vi "MIPI_RFEE_Create Patterns and save to HWS file_Wo_SetID.vi"(1 "Write Data":cluster{"USID":u8, "Register":u8, "Data":u8} {"Register" format="%.0x"; "USID" max=15 format="%.0x"}, 2 "Mode":enum16{"Write", "Read"}(ring), 5 "file path":path=path "C:/Users/user/Documents/AD2240/Waveforms/RFFE6", 12 "Save .HWS?":bool, 13 "Filename":string) -> ()   [LabVIEW 2013]
doc: "This VI demonstaits how to write to and read back data from a MIPI device. To run this VI:\n1) Change Resource name to the name of your HSDIO card\n2) The MIPI clock will run at <Sample Clock Rate>/<Oversample Factor>. This is 26 MHz (full rate). If your device should be run at a slower rate, decrease the sample clock rate and (or) increase the oversample rate.\n3. At 104MHz, the RTD value should be ~5 for a 1.5 meter cable. If you are running at a different clock rate or using a different length cable, adjust the RTD Compensation value so the MIPI data is stable at the falling edge of the clock. If you need futher timing adjustment, consider setting the data position to \"Delay from Sample Clock Rising Edge\" and configuring this delay."
uses:
  MIPI_RFFE/Ctrls/RegReadWrite.ctl
  MIPI_RFFE/Ctrls/Configuration.ctl
  MIPI_RFFE/Ctrls/ClockDataChannels.ctl
  MIPI_RFFE/Ctrls/ExtendedRegReadWrite.ctl
panel:
  out "Digital Waveform Graph":digitalwaveform(graph)={"t0"=timestamp(3585852840.1106524 s since 1904-01-01), "dt"=5e-07, "Y"={"transitions"=[], "data"=[[1, 0, 1, 0], [1, 0, 1, 0], [1, 0, 1, 0], [1, 0, 1, 0], [1, 0, 1, 0], [1, 0, 1, 0], [1, 0, 1, 0], [1, 0, 1, 0], [0, 0, 0, 0], [0, 0, 0, 0], [0, 0, 0, 0], [0, 0, 0, 0], [0, 0, 0, 0], [0, 0, 0, 0], [0, 0, 0, 0], [0, 0, 0, 0], [0, 1, 0, 1], [0, 1, 0, 1], [0, 1, 0, 1], [0, 1, 0, 1], [0, 0, 0, 0], [0, 0, 0, 0], [0, 0, 0, 0], [0, 0, 0, 0], [1, 1, 1, 1], [1, 1, 1, 1], [1, 1, 1, 1], [1, 1, 1, 1], [1, 0, 1, 0], [1, 0, 1, 0], [1, 0, 1, 0], [1, 0, 1, 0], [1, 1, 1, 1], [1, 1, 1, 1], [1, 1, 1, 1], [1, 1, 1, 1], [1, 0, 1, 0], [1, 0, 1, 0], [1, 0, 1, 0], [1, 0, 1, 0], [0, 1, 0, 1], [0, 1, 0, 1], [0, 1, 0, 1], [0, 1, 0, 1], [0, 0, 0, 0], [0, 0, 0, 0], [0, 0, 0, 0], [0, 0, 0, 0], [0, 1, 0, 1], [0, 1, 0, 1], [0, 1, 0, 1], [0, 1, 0, 1], [0, 0, 0, 0], [0, 0, 0, 0], [0, 0, 0, 0], [0, 0, 0, 0], [1, 1, 1, 1], [1, 1, 1, 1], [1, 1, 1, 1], [1, 1, 1, 1], [1, 0, 1, 0], [1, 0, 1, 0], [1, 0, 1, 0], [1, 0, 1, 0], [0, 1, 0, 1], [0, 1, 0, 1], [0, 1, 0, 1], [0, 1, 0, 1], [0, 0, 0, 0], [0, 0, 0, 0], [0, 0, 0, 0], [0, 0, 0, 0], [1, 1, 1, 1], [1, 1, 1, 1], [1, 1, 1, 1], [1, 1, 1, 1], [1, 0, 1, 0], [1, 0, 1, 0], [1, 0, 1, 0], [1, 0, 1, 0], [1, 1, 1, 1], [1, 1, 1, 1], [1, 1, 1, 1], [1, 1, 1, 1], [1, 0, 1, 0], [1, 0, 1, 0], [1, 0, 1, 0], [1, 0, 1, 0], [1, 1, 1, 1], [1, 1, 1, 1], [1, 1, 1, 1], [1, 1, 1, 1], [1, 0, 1, 0], [1, 0, 1, 0], [1, 0, 1, 0], [1, 0, 1, 0], [0, 1, 0, 1], [0, 1, 0, 1], [0, 1, 0, 1], [0, 1, 0, 1], [0, 0, 0, 0], [0, 0, 0, 0], [0, 0, 0, 0], [0, 0, 0, 0], [0, 1, 0, 1], [0, 1, 0, 1], [0, 1, 0, 1], [0, 1, 0, 1], [0, 0, 0, 0], [0, 0, 0, 0], [0, 0, 0, 0], [0, 0, 0, 0], [1, 1, 1, 1], [1, 1, 1, 1], [1, 1, 1, 1], [1, 1, 1, 1], [1, 0, 1, 0], [1, 0, 1, 0], [1, 0, 1, 0], [1, 0, 1, 0], [1, 1, 1, 1], [1, 1, 1, 1], [1, 1, 1, 1], [1, 1, 1, 1], [1, 0, 1, 0], [1, 0, 1, 0], [1, 0, 1, 0], [1, 0, 1, 0], [0, 1, 0, 1], [0, 1, 0, 1], [0, 1, 0, 1], [0, 1, 0, 1], [0, 0, 0, 0], [0, 0, 0, 0], [0, 0, 0, 0], [0, 0, 0, 0], [0, 1, 0, 1], [0, 1, 0, 1], [0, 1, 0, 1], [0, 1, 0, 1], [0, 0, 0, 0], [0, 0, 0, 0], [0, 0, 0, 0], [0, 0, 0, 0], [0, 1, 0, 1], [0, 1, 0, 1], [0, 1, 0, 1], [0, 1, 0, 1], [0, 0, 0, 0], [0, 0, 0, 0], [0, 0, 0, 0], [0, 0, 0, 0], [0, 1, 0, 1], [0, 1, 0, 1], [0, 1, 0, 1], [0, 1, 0, 1], [0, 0, 0, 0], [0, 0, 0, 0], [0, 0, 0, 0], [0, 0, 0, 0], [0, 1, 0, 1], [0, 1, 0, 1], [0, 1, 0, 1], [0, 1, 0, 1], [0, 0, 0, 0], [0, 0, 0, 0], [0, 0, 0, 0], [0, 0, 0, 0], [0, 1, 0, 1], [0, 1, 0, 1], [0, 1, 0, 1], [0, 1, 0, 1], [0, 0, 0, 0], [0, 0, 0, 0], [0, 0, 0, 0], [0, 0, 0, 0], [0, 1, 0, 1], [0, 1, 0, 1], [0, 1, 0, 1], [0, 1, 0, 1], [0, 0, 0, 0], [0, 0, 0, 0], [0, 0, 0, 0], [0, 0, 0, 0], [0, 1, 0, 1], [0, 1, 0, 1], [0, 1, 0, 1], [0, 1, 0, 1], [0, 0, 0, 0], [0, 0, 0, 0], [0, 0, 0, 0], [0, 0, 0, 0], [0, 1, 0, 1], [0, 1, 0, 1], [0, 1, 0, 1], [0, 1, 0, 1], [0, 0, 0, 0], [0, 0, 0, 0], [0, 0, 0, 0], [0, 0, 0, 0], [1, 0, 1, 0], [1, 0, 1, 0], [1, 0, 1, 0], [1, 0, 1, 0], [1, 0, 1, 0], [1, 0, 1, 0], [1, 0, 1, 0], [1, 0, 1, 0], [0, 0, 0, 0], [0, 0, 0, 0], [0, 0, 0, 0], [0, 0, 0, 0], [0, 0, 0, 0], [0, 0, 0, 0], [0, 0, 0, 0], [0, 0, 0, 0], [0, 1, 0, 1], [0, 1, 0, 1], [0, 1, 0, 1], [0, 1, 0, 1], [0, 0, 0, 0], [0, 0, 0, 0], [0, 0, 0, 0], [0, 0, 0, 0], [1, 1, 1, 1], [1, 1, 1, 1], [1, 1, 1, 1], [1, 1, 1, 1], [1, 0, 1, 0], [1, 0, 1, 0], [1, 0, 1, 0], [1, 0, 1, 0], [1, 1, 1, 1], [1, 1, 1, 1], [1, 1, 1, 1], [1, 1, 1, 1], [1, 0, 1, 0], [1, 0, 1, 0], [1, 0, 1, 0], [1, 0, 1, 0], [0, 1, 0, 1], [0, 1, 0, 1], [0, 1, 0, 1], [0, 1, 0, 1], [0, 0, 0, 0], [0, 0, 0, 0], [0, 0, 0, 0], [0, 0, 0, 0], [0, 1, 0, 1], [0, 1, 0, 1], [0, 1, 0, 1], [0, 1, 0, 1], [0, 0, 0, 0], [0, 0, 0, 0], [0, 0, 0, 0], [0, 0, 0, 0], [1, 1, 1, 1], [1, 1, 1, 1], [1, 1, 1, 1], [1, 1, 1, 1], [1, 0, 1, 0], [1, 0, 1, 0], [1, 0, 1, 0], [1, 0, 1, 0], [1, 1, 1, 1], [1, 1, 1, 1], [1, 1, 1, 1], [1, 1, 1, 1], [1, 0, 1, 0], [1, 0, 1, 0], [1, 0, 1, 0], [1, 0, 1, 0], [1, 1, 1, 1], [1, 1, 1, 1], [1, 1, 1, 1], [1, 1, 1, 1], [1, 0, 1, 0], [1, 0, 1, 0], [1, 0, 1, 0], [1, 0, 1, 0], [1, 1, 1, 1], [1, 1, 1, 1], [1, 1, 1, 1], [1, 1, 1, 1], [1, 0, 1, 0], [1, 0, 1, 0], [1, 0, 1, 0], [1, 0, 1, 0], [1, 1, 1, 1], [1, 1, 1, 1], [1, 1, 1, 1], [1, 1, 1, 1], [1, 0, 1, 0], [1, 0, 1, 0], [1, 0, 1, 0], [1, 0, 1, 0], [0, 1, 0, 1], [0, 1, 0, 1], [0, 1, 0, 1], [0, 1, 0, 1], [0, 0, 0, 0], [0, 0, 0, 0], [0, 0, 0, 0], [0, 0, 0, 0], [0, 1, 0, 1], [0, 1, 0, 1], [0, 1, 0, 1], [0, 1, 0, 1], [0, 0, 0, 0], [0, 0, 0, 0], [0, 0, 0, 0], [0, 0, 0, 0], [0, 1, 0, 1], [0, 1, 0, 1], [0, 1, 0, 1], [0, 1, 0, 1], [0, 0, 0, 0], [0, 0, 0, 0], [0, 0, 0, 0], [0, 0, 0, 0], [0, 1, 0, 1], [0, 1, 0, 1], [0, 1, 0, 1], [0, 1, 0, 1], [0, 0, 0, 0], [0, 0, 0, 0], [0, 0, 0, 0], [0, 0, 0, 0], [1, 1, 5, 1], [1, 1, 5, 1], [1, 1, 5, 1], [1, 1, 5, 1], [1, 0, 4, 0], [1, 0, 5, 0], [1, 0, 5, 0], [1, 0, 5, 0], [0, 1, 5, 1], [0, 1, 5, 1], [0, 1, 5, 1], [0, 1, 5, 1], [0, 0, 3, 0], [0, 0, 5, 0], [0, 0, 5, 0], [0, 0, 5, 0], [0, 1, 5, 1], [0, 1, 5, 1], [0, 1, 5, 1], [0, 1, 5, 1], [0, 0, 3, 0], [0, 0, 5, 0], [0, 0, 5, 0], [0, 0, 5, 0], [0, 1, 5, 1], [0, 1, 5, 1], [0, 1, 5, 1], [0, 1, 5, 1], [0, 0, 3, 0], [0, 0, 5, 0], [0, 0, 5, 0], [0, 0, 5, 0], [0, 1, 5, 1], [0, 1, 5, 1], [0, 1, 5, 1], [0, 1, 5, 1], [0, 0, 3, 0], [0, 0, 5, 0], [0, 0, 5, 0], [0, 0, 5, 0], [0, 1, 5, 1], [0, 1, 5, 1], [0, 1, 5, 1], [0, 1, 5, 1], [0, 0, 3, 0], [0, 0, 5, 0], [0, 0, 5, 0], [0, 0, 5, 0], [0, 1, 5, 1], [0, 1, 5, 1], [0, 1, 5, 1], [0, 1, 5, 1], [0, 0, 3, 0], [0, 0, 5, 0], [0, 0, 5, 0], [0, 0, 5, 0], [0, 1, 5, 1], [0, 1, 5, 1], [0, 1, 5, 1], [0, 1, 5, 1], [0, 0, 3, 0], [0, 0, 5, 0], [0, 0, 5, 0], [0, 0, 5, 0], [0, 1, 5, 1], [0, 1, 5, 1], [0, 1, 5, 1], [0, 1, 5, 1], [0, 0, 3, 0], [0, 0, 5, 0], [0, 0, 5, 0], [0, 0, 5, 0], [0, 1, 0, 1], [0, 1, 0, 1], [0, 1, 0, 1], [0, 1, 0, 1], [0, 0, 0, 0], [0, 0, 0, 0], [0, 0, 0, 0], [0, 0, 0, 0]]}}
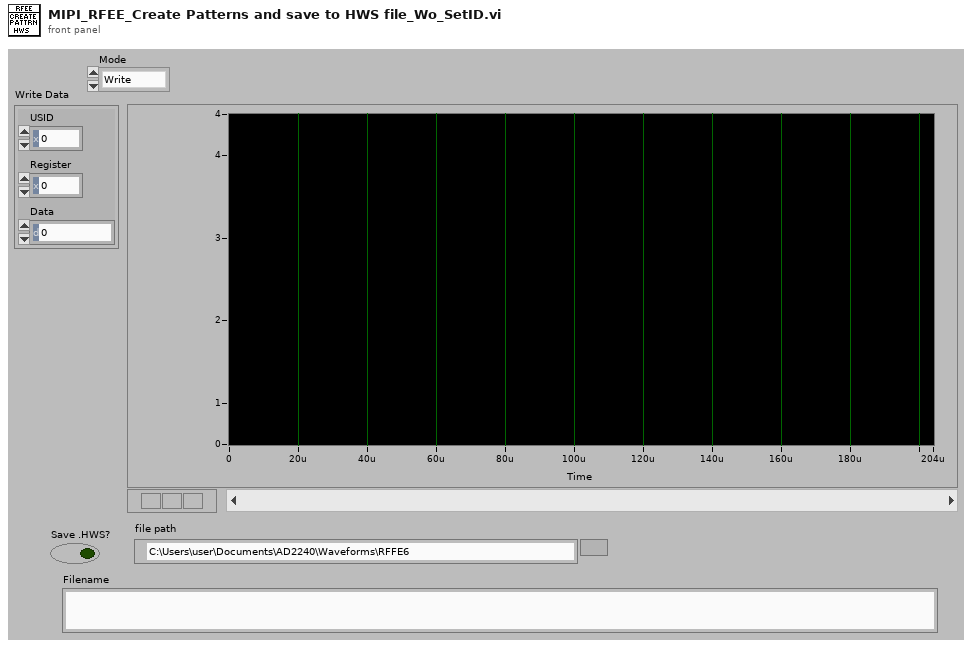
[diagram p1: front panel]
types:
  T1 = typedef "Configuration.ctl" = cluster{"Samples to Allocate":i32, "Oversample Factor":u8, "Clock Channel":T2, "Data Channel":T2}
  T2 = typedef "ClockDataChannels.ctl" = enum16{"0", "1"}
  T3 = typedef "RegReadWrite.ctl" = cluster{"Slave Address":u8, "Register":u8, "Data":u8, "SetID_Pin_State":enum16{"0", "1", "Z"}}
  T4 = typedef "RFFE_Data.ctl" = cluster{"Clock Channel":T2, "Data Channel":T2, "Oversample Factor":u8, "Zero Array":u8[], "One Array":u8[], "Z Array ":u8[], "H Array":u8[], "L Array":u8[], "X Array":u8[], "Toggle (high to low)":u8[]}
  T5 = typedef "ExtendedRegReadWrite.ctl" = cluster{"Slave Address":u8, "Register":u8, "Data":u8[]}
  T6 = typedef "ReadInfo.ctl" = cluster{"Expected Value(s)":u8[], "Compare Locations":u32[]}
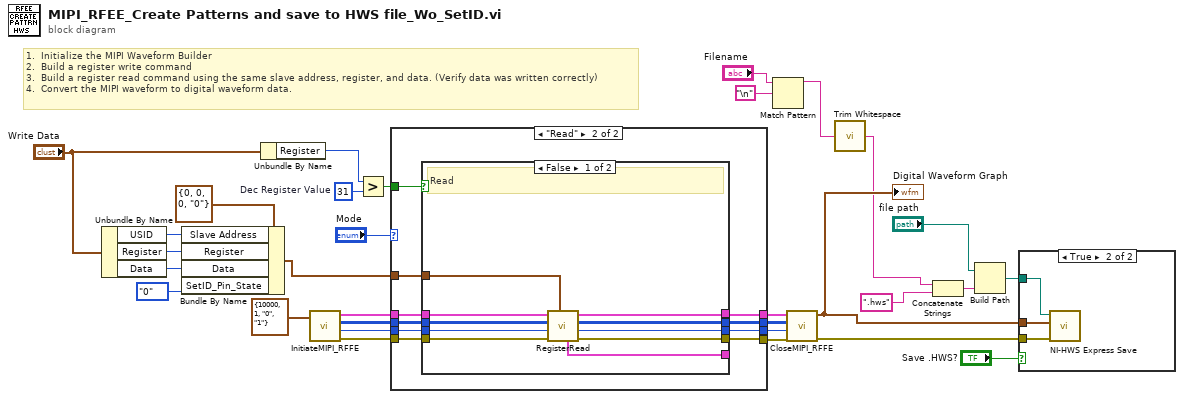
[diagram p0: block diagram]
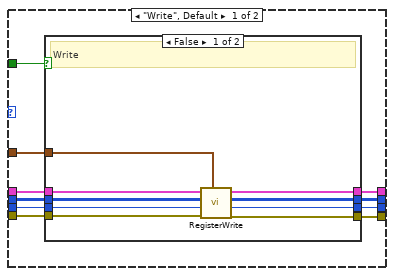
[diagram p2: hidden frame]
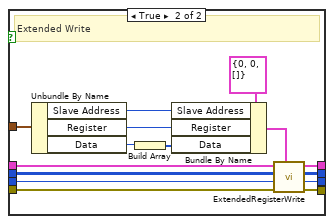
[diagram p3: hidden frame]
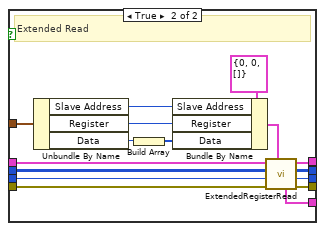
[diagram p4: hidden frame]
diagram:
  w27 = u8 31  # Dec Register Value
  # "1.  Initialize the MIPI Waveform Builder\n2.  Build a register write command\n3.  Build a register read command using the same slave address, register, and data. (Verify data was written correctly)\n4.  Convert the MIPI waveform to digital waveform data."
  n1 = Unbundle By Name("Write Data") -> ("USID"=w9:u8, "Register"=w11:u8, "Data"=w10:u8)
  n2 = Bundle By Name(cluster=T3 {"Slave Address"=0, "Register"=0, "Data"=0, "SetID_Pin_State"=enum."0"} ("Write Data"), "Slave Address"=w9, "Register"=w11, "Data"=w10, "SetID_Pin_State"=enum16{"0", "1", "Z"}."0") -> (w7:T3)
  n3 = Unbundle By Name("Write Data") -> ("Register"=w26:u8)
  n4 = call "InitiateMIPI_RFFE.vi"("Configuratation In"=T1 {"Samples to Allocate"=10000, "Oversample Factor"=1, "Clock Channel"=enum."0", "Data Channel"=enum."1"} ("Configuratation")) -> ("error out"=w31:errorcluster, "Number of Samples Out"=w30:i32, "Data Array"=w29:u8[][], "RFFE_Data"=w28:T4)  [unwired: 7 in]
  n5 = Greater?(x=w26, y=w27) -> (0:w25:bool)
  n6 = case shown="\"Read\"" "Mode" {
    tunnel: w31 -> [w41 w74]
    tunnel: w30 -> [w40 w71]
    tunnel: w29 -> [w39 w72]
    tunnel: w28 -> [w38 w73]
    tunnel: w7 -> [w37 w66]
    tunnel: w25 -> [w36 w75]
    tunnel: [w35 w67] -> w24
    tunnel: [w34 w68] -> w23
    tunnel: [w33 w70] -> w14
    tunnel: [w32 w69] -> w19
    frame "Write", Default {
      n7 = case shown="False" w36 {
        tunnel: w41 -> [w50 w65]
        tunnel: w40 -> [w49 w62]
        tunnel: w39 -> [w48 w63]
        tunnel: w38 -> [w47 w64]
        tunnel: w37 -> [w42 w60]
        tunnel: [w46 w54] -> w35
        tunnel: [w45 w53] -> w34
        tunnel: [w44 w52] -> w33
        tunnel: [w43 w51] -> w32
        frame False {
          # "Write"
          n8 = call "RegisterWrite.vi"("Write Data"=w42, "error in (no error)"=w50, "Number of Samples In"=w49, "Data Array"=w48, "RFFE_Data"=w47) -> ("error out"=w43:errorcluster, "Number of Samples Out"=w44:i32, "Data Array Out"=w45:u8[][], "Configuratation Out"=w46:T4)  [unwired: 3 in]
        }
        frame True {
          # "Extended Write"
          n9 = Unbundle By Name(w60) -> ("Slave Address"=w59:u8, "Register"=w58:u8, "Data"=w57:u8)
          n10 = Build Array(w57) -> (w56:u8[])
          n11 = Bundle By Name(cluster=T5 {"Slave Address"=0, "Register"=0, "Data"=[]} ("Extended Read/Write"), "Slave Address"=w59, "Register"=w58, "Data"=w56) -> (w55:T5)
          n12 = call "ExtendedRegisterWrite.vi"("Extended Read/Write"=w55, "error in (no error)"=w65, "Number of Samples In"=w62, "Data Array"=w63, "RFFE_Data In"=w64) -> ("error out"=w51:errorcluster, "Number of Samples Out"=w52:i32, "Data Array Out"=w53:u8[][], "RFFE_Data Out"=w54:T4)  [unwired: 3 in]
        }
      }
    }
    frame "Read" {
      n13 = case shown="False" w75 {
        tunnel: [w85 w96] -> w67
        tunnel: [w84 w97] -> w68
        tunnel: [w83 w98] -> w70
        tunnel: [w82 w99] -> w69
        tunnel: [w81 w94] -> _
        tunnel: w74 -> [w80 w86]
        tunnel: w73 -> [w79 w89]
        tunnel: w72 -> [w78 w88]
        tunnel: w71 -> [w77 w87]
        tunnel: w66 -> [w76 w93]
        frame False {
          # "Read"
          n14 = call "RegisterRead.vi"("Register Read/Write"=w76, "error in (no error)"=w80, "Number of Samples In"=w77, "Data Array"=w78, "RFFE_Data In"=w79) -> ("error out"=w82:errorcluster, "Number of Samples Out out"=w83:i32, "Data Array Out"=w84:u8[][], "RFFE_Data Out"=w85:T4, "Compare Bits Out"=w81:T6[])  [unwired: 2 in]
        }
        frame True {
          # "Extended Read"
          n15 = Unbundle By Name(w93) -> ("Slave Address"=w91:u8, "Register"=w92:u8, "Data"=w100:u8)
          n16 = Build Array(w100) -> (w90:u8[])
          n17 = Bundle By Name(cluster=T5 {"Slave Address"=0, "Register"=0, "Data"=[]} ("Extended Read/Write"), "Slave Address"=w91, "Register"=w92, "Data"=w90) -> (w95:T5)
          n18 = call "ExtendedRegisterRead.vi"("Extended Read/Write"=w95, "error in (no error)"=w86, "Number of Samples In"=w87, "Data Array"=w88, "RFFE_Data In"=w89) -> ("error out"=w99:errorcluster, "Number of Samples Out out"=w98:i32, "Data Array Out"=w97:u8[][], "RFFE_Data Out"=w96:T4, "Compare Bits Out"=w94:T6[])  [unwired: 2 in]
        }
      }
    }
  }
  n19 = Match Pattern(string="Filename", regular expression="\n") -> (before substring=w1:string)  [unwired: 1 in, 3 out]
  n20 = call "CloseMIPI_RFFE.vi"("error in (no error)"=w19, "Number of Samples"=w14, "Data Array"=w23, "RFFE_Data"=w24) -> ("error out"=w6:errorcluster, "Digital Waveform"=w5:digitalwaveform)  [unwired: 6 in]
  "Digital Waveform Graph" <- w5
  n21 = call <vilib>:"Trim Whitespace.vi"("string"=w1) -> ("trimmed string"=w4:string)  [unwired: 1 in]
  n22 = Concatenate Strings(w4, ".hws" ("string")) -> (w16:string)
  n23 = Build Path(base path="file path", name or relative path=w16) -> (appended path=w20:path)
  n24 = case shown="True" "Save .HWS?" {
    tunnel: w20 -> [_ w104]
    tunnel: w6 -> [_ w103]
    tunnel: w5 -> [_ w102]
    frame False {
    }
    frame True {
      n25 = call "NI-HWS Express Save"("error in"=w103, "digital waveform"=w102, "file path"=w104) -> ()  [unwired: 8 in, 1 out]
    }
  }
